vi "NF87xx.evt call Relative Move.vi"(0 "i ref in":refnum<vi>, 1 "Instance":string="N/A", 2 "Motor (0, 1 or 2)":i32, 3 "steps":i32, 4 "velocity (10 .. 2000)":dbl=10.0 min=10.0 max=2000.0, 5 "error in (no error)":errorcluster, 6 "System":string="N/A", 7 "acceleration (20000)":dbl=20000.0 min=16.0 max=20000.0, 9 "start velocity (8)":dbl=8.0 min=0.0 max=1999.0) -> (14 "i ref out":refnum<vi>, 19 "error out":errorcluster)   [LabVIEW 2014, in "NF87XX.lvlib"]
doc: "This VI sets the \"RelMove\" case by a notification call. The instance has to be something else but N/A and the Motor 0, 1 or 2. Steps has to be more than 0, negavie values are allowed (the direction is defined by that). The parameter are corced to the allowed range."
uses:
  NF87XX.lvlib
  CS_Core/CSSystem/CoreLib/CoreLib.double 2 byte array.vi
  CS_Core/CSSystem/CoreLib/CoreLib.int 2 byte array.vi
  CS_Core/CSSystem/CoreLib/CoreLib.string 2 byte array.vi
  CS_Core/BaseProcess/BaseProcess.lvlib
  CS_Core/CSSystem/CoreLib/CoreLib.lvlib
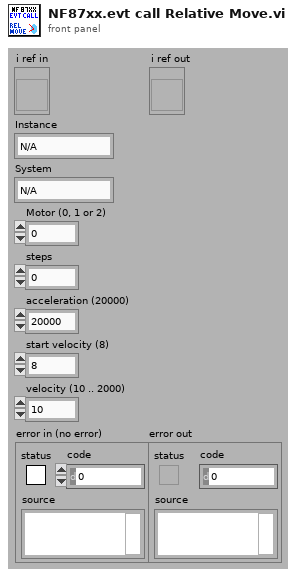
[diagram p1: front panel]
types:
  T1 = enum16{"simple", "synchronous", "asynchronous", "notification"}
  T2 = typedef "CoreDefs.rawDataType.ctl" = i8[]
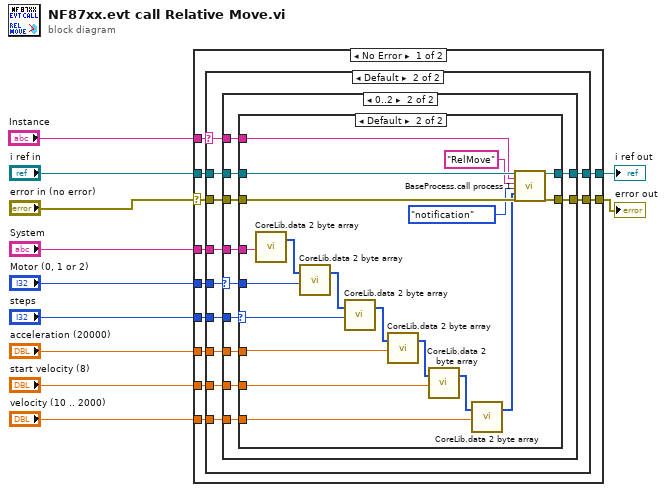
[diagram p0: block diagram]
diagram:
  n1 = case shown="No Error" "error in (no error)" {
    selector: "error in (no error)" -> [w13 w70]
    tunnel: [w22 w71] -> w11
    tunnel: [w21 w70] -> w10
    tunnel: "i ref in" -> [w20 w71]
    tunnel: "Motor (0, 1 or 2)" -> [w19 _]
    tunnel: "velocity (10 .. 2000)" -> [w18 _]
    tunnel: "start velocity (8)" -> [w17 _]
    tunnel: "acceleration (20000)" -> [w16 _]
    tunnel: "steps" -> [w15 _]
    tunnel: "Instance" -> [w14 _]
    tunnel: "System" -> [w12 _]
    frame No Error {
      n2 = case shown="Default" w14 {
        selector: w14 -> [_ w27]
        tunnel: [w24 w35] -> w22
        tunnel: [w23 w34] -> w21
        tunnel: w20 -> [w24 w33]
        tunnel: w13 -> [w23 w32]
        tunnel: w19 -> [_ w26]
        tunnel: w18 -> [_ w31]
        tunnel: w17 -> [_ w30]
        tunnel: w16 -> [_ w29]
        tunnel: w15 -> [_ w28]
        tunnel: w12 -> [_ w25]
        frame "N/A" {
        }
        frame Default {
          n3 = case shown="0..2" w26 {
            selector: w26 -> [_ w40]
            tunnel: [w36 w48] -> w35
            tunnel: [w37 w47] -> w34
            tunnel: w33 -> [w36 w46]
            tunnel: w32 -> [w37 w45]
            tunnel: w31 -> [_ w44]
            tunnel: w30 -> [_ w43]
            tunnel: w29 -> [_ w42]
            tunnel: w28 -> [_ w39]
            tunnel: w27 -> [_ w41]
            tunnel: w25 -> [_ w38]
            frame Default {
            }
            frame 0..2 {
              n4 = case shown="Default" w39 {
                selector: w39 -> [_ w62]
                tunnel: [w50 w69] -> w48
                tunnel: [w49 w68] -> w47
                tunnel: w46 -> [w50 w67]
                tunnel: w45 -> [w49 w66]
                tunnel: w44 -> [_ w53]
                tunnel: w43 -> [_ w57]
                tunnel: w42 -> [_ w58]
                tunnel: w41 -> [_ w63]
                tunnel: w40 -> [_ w61]
                tunnel: w38 -> [_ w52]
                frame 0 {
                }
                frame Default {
                  n5 = call-poly "CoreLib.data 2 byte array.vi"("string"=w52) -> ("byteArray out"=w51:T2)  [unwired: 18 in]
                  n6 = call-poly "CoreLib.data 2 byte array.vi"("byteArray"=w51, "i32"=w61) -> ("byteArray out"=w60:T2)  [unwired: 17 in]
                  n7 = call-poly "CoreLib.data 2 byte array.vi"("byteArray"=w60, "i32"=w62) -> ("byteArray out"=w59:T2)  [unwired: 17 in]
                  n8 = call-poly "CoreLib.data 2 byte array.vi"("byteArray"=w59, "f64"=w58) -> ("byteArray out"=w56:T2)  [unwired: 17 in]
                  n9 = call-poly "CoreLib.data 2 byte array.vi"("byteArray"=w56, "f64"=w57) -> ("byteArray out"=w54:T2)  [unwired: 17 in]
                  n10 = call-poly "CoreLib.data 2 byte array.vi"("byteArray"=w54, "f64"=w53) -> ("byteArray out"=w55:T2)  [unwired: 17 in]
                  n11 = call "BaseProcess.call process 1.vi"("i ref in"=w67, "Object"=w63, "Selector"="RelMove", "CallType"=T1."notification", "Data"=w55, "error in (no error)"=w66) -> ("i ref out"=w69:refnum<vi>, "error out"=w68:errorcluster)  [unwired: 11 in, 1 out]
                }
              }
            }
          }
        }
      }
    }
    frame Error {
    }
  }
  "error out" <- w10
  "i ref out" <- w11
